vi "ClimberManualJoystickControl.vi"(0 "Joystick control":T2, 1 "OperatorControlBox Buttons":T1, 2 "OperatorControlBoxConnected":bool) -> (3 "FrontClimb":dbl, 4 "RearClimb":dbl, 5 "ClimbDrive":dbl, 6 "Auto Climb Start":bool)   [LabVIEW 2018]
uses:
  TypeDefs/JoystickControls.ctl
  General/OperatorControlBox/TypeDefs/OperatorControlBoxButtons_Type.ctl
  ArgosLib/ArgosLib.lvlib
panel:
  in  "AutoClimbCtrlDebounce (ms)":u32=1000
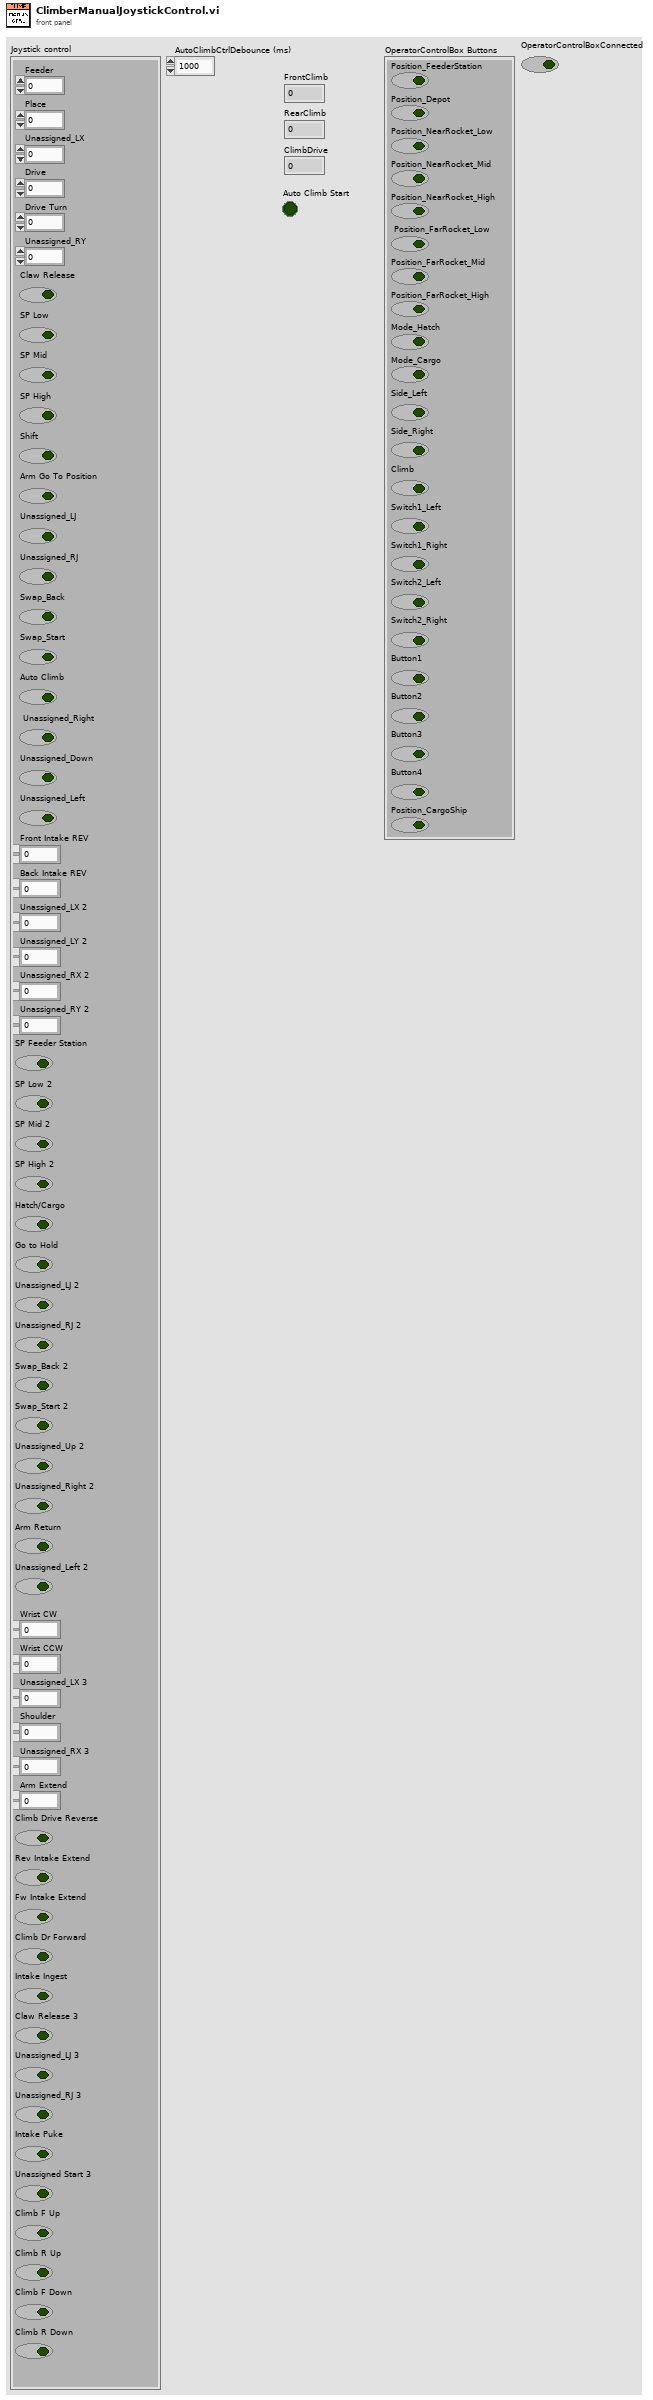
[diagram p1: front panel]
types:
  T1 = typedef "OperatorControlBoxButtons_Type.ctl" = cluster{"Position_FeederStation":bool, "Position_Depot":bool, "Position_NearRocket_Low":bool, "Position_NearRocket_Mid":bool, "Position_NearRocket_High":bool, " Position_FarRocket_Low":bool, "Position_FarRocket_Mid":bool, "Position_FarRocket_High":bool, "Mode_Hatch":bool, "Mode_Cargo":bool, "Side_Left":bool, "Side_Right":bool, "Climb":bool, "Switch1_Left":bool, "Switch1_Right":bool, "Switch2_Left":bool, "Switch2_Right":bool, "Button1":bool, "Button2":bool, "Button3":bool, "Button4":bool, "Position_CargoShip":bool}
  T2 = typedef "JoystickControls.ctl" = cluster{"Drive":dbl, "Drive Turn ":dbl, "Unassigned_LX":dbl, "Unassigned_RY":dbl, "Claw Release":bool, "Place":dbl, "Feeder":dbl, "SP Low":bool, "SP Mid":bool, "SP High":bool, "Shift":bool, "Arm Go To Position":bool, "Unassigned_LJ":bool, "Unassigned_RJ":bool, "Swap_Back":bool, "Swap_Start":bool, "Unassigned_LY 2":dbl, "Unassigned_RX 2":dbl, "Unassigned_LX 2":dbl, "Unassigned_RY 2":dbl, "SP Feeder Station":bool, "Back Intake REV":dbl, "Front Intake REV":dbl, "SP Low 2":bool, "SP Mid 2":bool, "SP High 2":bool, "Hatch/Cargo":bool, "Go to Hold":bool, "Unassigned_LJ 2":bool, "Unassigned_RJ 2":bool, "Swap_Back 2":bool, "Swap_Start 2":bool, "Unassigned_Up 2":bool, "Unassigned_Right 2":bool, "Arm Return":bool, "Unassigned_Left 2":bool, "Auto Climb":bool, " Unassigned_Right":bool, "Unassigned_Down":bool, "Unassigned_Left":bool, "Shoulder":dbl, "Unassigned_RX 3":dbl, "Unassigned_LX 3":dbl, "Arm Extend":dbl, "Climb Drive Reverse":bool, "Wrist CCW":dbl, "Wrist CW":dbl, "Rev Intake Extend":bool, "Fw Intake Extend":bool, "Climb Dr Forward":bool, "Intake Ingest ":bool, "Claw Release 3":bool, "Unassigned_LJ 3":bool, "Unassigned_RJ 3":bool, "Intake Puke":bool, "Unassigned Start 3":bool, "Climb F Up":bool, "Climb R Up":bool, "Climb F Down":bool, "Climb R Down":bool}
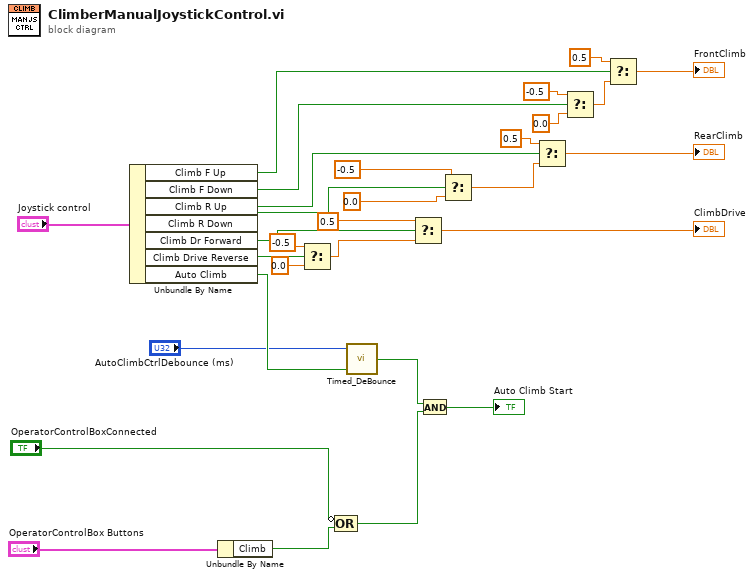
[diagram p0: block diagram]
diagram:
  n1 = Unbundle By Name("Joystick control") -> ("Climb F Up"=w25:bool, "Climb F Down"=w26:bool, "Climb R Up"=w27:bool, "Climb R Down"=w28:bool, "Climb Dr Forward"=w29:bool, "Climb Drive Reverse"=w30:bool, "Auto Climb"=w8:bool)
  n2 = Unbundle By Name("OperatorControlBox Buttons") -> ("Climb"=w5:bool)
  n3 = Select(t=-0.5, s=w30, f=0.0) -> (s? t:f=w24:dbl)
  n4 = Compound Arithmetic op=OR(invert "OperatorControlBoxConnected", w5) -> (w3:bool)
  n5 = call "Timed_DeBounce.vi"("Input"=w8, "Hold Time(ms)"="AutoClimbCtrlDebounce (ms)") -> ("Output"=w2:bool)  [unwired: 1 in]
  n6 = Select(t=0.5, s=w29, f=w24) -> (s? t:f=→"ClimbDrive":dbl)
  n7 = And(x=w2, y=w3) -> (x .and. y?=→"Auto Climb Start":bool)
  n8 = Select(t=-0.5, s=w28, f=0.0) -> (s? t:f=w23:dbl)
  n9 = Select(t=0.5, s=w27, f=w23) -> (s? t:f=→"RearClimb":dbl)
  n10 = Select(t=-0.5, s=w26, f=0.0) -> (s? t:f=w22:dbl)
  n11 = Select(t=0.5, s=w25, f=w22) -> (s? t:f=→"FrontClimb":dbl)
